vi "Level2Copy.vi"(8 "error in (no error)":errorcluster, 11 "TheConsumer in":refnum<class "TheConsumer.lvclass">) -> (0 "error out":errorcluster, 1 "BaseClassDependency out":refnum<class "BaseClassDependency.lvclass">, 2 "Level1Class out":refnum<class "Level1Class.lvclass">, 3 "TheConsumer out":refnum<class "TheConsumer.lvclass">)   [LabVIEW 2019, in "TheConsumer.lvlib" / "TheConsumer.lvclass"]
uses:
  TheConsumer.lvclass
  ALevel2ClassCopy/ALevel2ClassCopy.lvclass
  Level1Class/Level1Class.lvclass
  BaseClassDependency/BaseClassDependency.lvclass
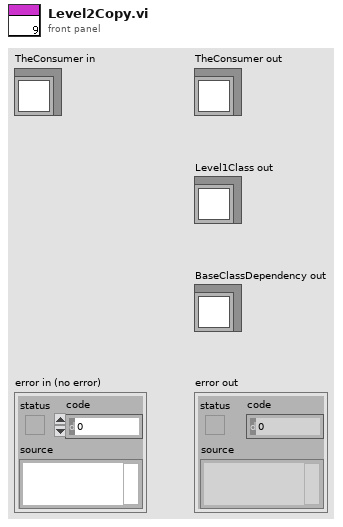
[diagram p1: front panel]
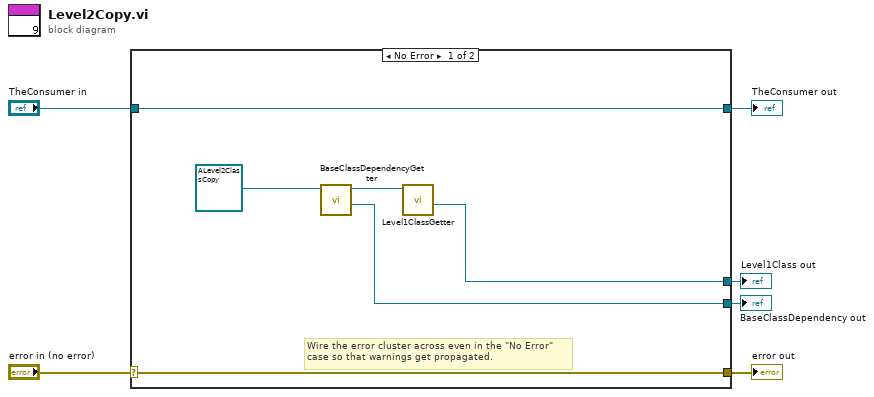
[diagram p0: block diagram]
diagram:
  n1 = case shown="No Error" "error in (no error)" {
    selector: "error in (no error)" -> [w11 w14]
    tunnel: [w11 w14] -> w5
    tunnel: [w12 w13] -> w3
    tunnel: "TheConsumer in" -> [w12 w13]
    tunnel: [w8 _] -> w1
    tunnel: [w7 _] -> w2
    frame No Error {
      # "Wire the error cluster across even in the \"No Error\"\ncase so that warnings get propagated."
      n2 = call-dynamic "BaseClassDependencyGetter.vi"("ALevel2ClassCopy in"=refnum<class "ALevel2ClassCopy.lvclass"> refnum ("ALevel2ClassCopy.lvlib:ALevel2ClassCopy.lvclass")) -> ("BaseClassDependency out"=w8:refnum<class "BaseClassDependency.lvclass">, "ALevel2ClassCopy out"=w9:refnum<class "ALevel2ClassCopy.lvclass">)  [unwired: 8 in, 1 out]
      n3 = call-dynamic "Level1ClassGetter.vi"("ALevel2ClassCopy in"=w9) -> ("Level1Class out"=w7:refnum<class "Level1Class.lvclass">)  [unwired: 8 in, 2 out]
    }
    frame Error {
    }
  }
  "error out" <- w5
  "TheConsumer out" <- w3
  "Level1Class out" <- w2
  "BaseClassDependency out" <- w1
